vi "rad_GetInstalledSoftware.vi"(8 "error in (no error)":errorcluster, 11 "Target settings":T1={"Hostname"="", "Serial number"="", "Product name"="", "Product code"=0, "System status"="", "Credential type"=enum."None/Unlocked", "User added?"=FALSE, "Primary NIC"={"MAC address"="", "IP Address Request Mode"=2, "IP address"="", "Subnet mask"="", "Gateway"="", "DNS server"=""}} {"Primary NIC"."IP Address Request Mode" items=["Static"=1, "DHCP/Link-Local"=2, "Link-Local Only"=4, "DHCP Only"=8]}) -> (0 "error out":errorcluster, 3 "installedSoftware":string[](array[string]))   [LabVIEW 2020]
uses:
  <vilib>/nisyscfg/nisyscfg.lvlib
  <vilib>/nisyscfg/Get Installed Components.vi
  <vilib>/nisyscfg/Close (System).vi
  Targets/TypeDefs/rad_Target Information.ctl
  Targets/TypeDefs/rad_Target Network Settings.ctl
panel:
  in  "Password":string
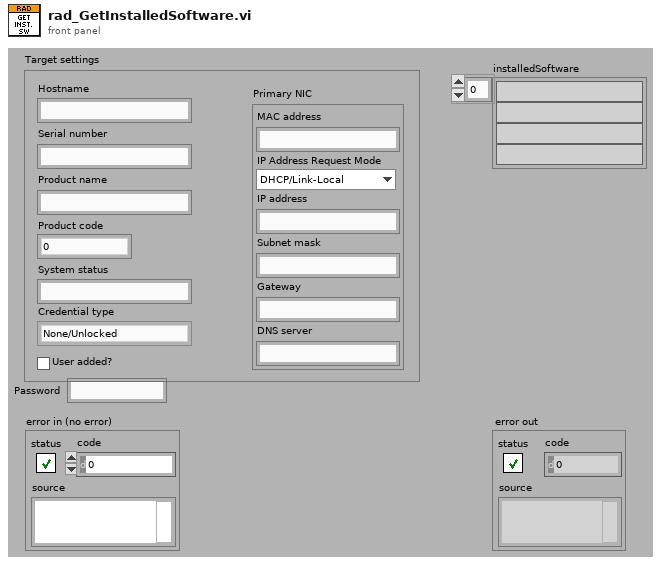
[diagram p1: front panel]
types:
  T1 = typedef "rad_Target Information.ctl" = cluster{"Hostname":string, "Serial number":string, "Product name":string, "Product code":i32, "System status":string, "Credential type":enum16{"None/Unlocked", "FTP Password", "NIAuth Credentials"}, "User added?":bool, "Primary NIC":T2}
  T2 = typedef "rad_Target Network Settings.ctl" = cluster{"MAC address":string, "IP Address Request Mode":i32, "IP address":string, "Subnet mask":string, "Gateway":string, "DNS server":string}
  T3 = typedef "nisyscfg.lvlib/Software 1.2.ctl" = cluster{"title":string, "description":string, "ID":string, "version":string, "component type":T4}
  T4 = typedef "nisyscfg.lvlib/Component Type.ctl" = u32
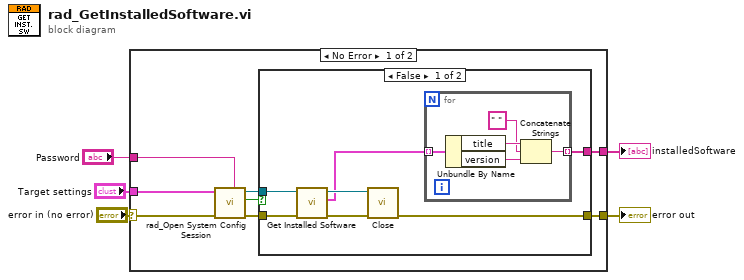
[diagram p0: block diagram]
diagram:
  n1 = case shown="No Error" "error in (no error)" {
    selector: "error in (no error)" -> [w11 w27]
    tunnel: [w13 w27] -> w5
    tunnel: [w12 _] -> w3
    tunnel: "Target settings" -> [w7 _]
    tunnel: "Password" -> [w6 _]
    frame No Error {
      n2 = call "rad_Open System Config Session.vi"("Password"=w6, "error in (no error)"=w11, "Target settings"=w7) -> ("error out"=w9:errorcluster, "Cancelled"=w8:bool, "Session out"=w10:refnum<k21>)  [unwired: 5 in, 1 out]
      n3 = case shown="False" w8 {
        tunnel: [w18 w26] -> w13
        tunnel: [w16 _] -> w12
        tunnel: w10 -> [w15 _]
        tunnel: w9 -> [w14 w26]
        frame False {
          n4 = call-poly <vilib>:"Get Installed Software.vi"("error in (no error)"=w14, "Session in"=w15) -> ("error out"=w20:errorcluster, "Software Components"=w17:T3[], "Session out"=w19:refnum<k21>)  [unwired: 7 in]
          n5 = call-poly <vilib>:"Close.vi"("error in (no error)"=w20, "Session in"=w19) -> ("error out"=w18:errorcluster)  [unwired: 9 in]
          n6 = for {
            tunnel: w17 -> [w25] mode=indexing
            tunnel: [w21] -> w16 mode=indexing
            n7 = Unbundle By Name(w25) -> ("title"=w24:string, "version"=w23:string)
            n8 = Concatenate Strings(w24, " " ("string"), w23) -> (w21:string)
          }
        }
        frame True {
        }
      }
    }
    frame Error {
    }
  }
  "error out" <- w5
  "installedSoftware" <- w3
